vi "UTIL Progress Bar ShowHide Abort.vi"(8 "error in (no error)":errorcluster, 10 "Show Abort":bool, 11 "reference in":refnum<vi>) -> (0 "error out":errorcluster, 3 "reference out":refnum<vi>)   [LabVIEW 2019]
doc: "10/01/2010\n\nNational Analytics (TLE)\n\nCause the Abort button to be visible."
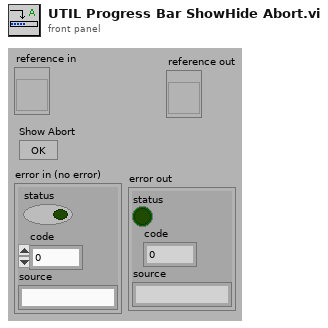
[diagram p1: front panel]
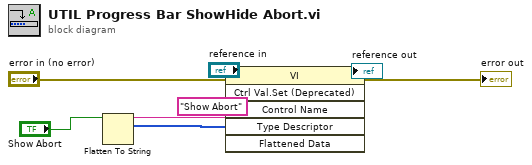
[diagram p0: block diagram]
diagram:
  n1 = Flatten To String(anything="Show Abort") -> (data string=w6:string, type string=w7:i16[])  [unwired: 1 in, 3 out]
  n2 = invoke class="VI" method="Ctrl Val.Set (Deprecated)"(reference="reference in", error in="error in (no error)", "Control Name"="Show Abort", "Type Descriptor"=w7, "Flattened Data"=w6) -> (reference out=→"reference out":refnum<vi>, error out=→"error out":errorcluster)  [unwired: 1 in, 4 out]
